vi "Obtain Module Semaphore.vi"(8 "error in":errorcluster) -> (0 "error out":errorcluster, 1 "created new?":bool, 3 "semaphore":T1)   [LabVIEW 2020, in "Camera Acquisition.lvlib"]
doc: "Obtain this module's Semaphore that locks down operations on the Clone Registry and VI Reference action engines.\n_____\nBased on DQMH Project Template 6.0.0.91."
uses:
  Camera Acquisition.lvlib
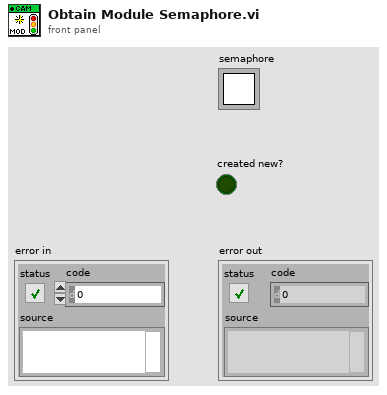
[diagram p1: front panel]
types:
  T1 = typedef "Semaphore RefNum" = refnum<k1>
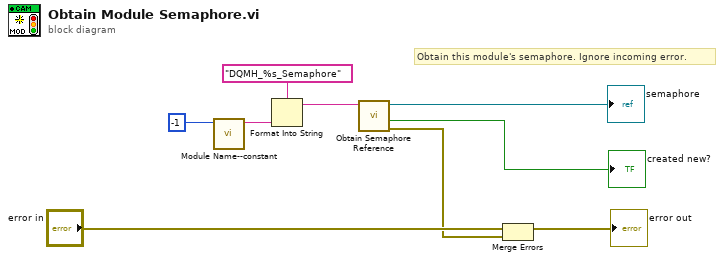
[diagram p0: block diagram]
diagram:
  # "Obtain this module's semaphore. Ignore incoming error."
  n1 = call "Module Name--constant.vi"("Module ID"=-1) -> ("Module Name"=w4:string)  [unwired: 10 in]
  n2 = Format Into String(format string="DQMH_%s_Semaphore", w4) -> (resulting string=w3:string)  [unwired: 2 in, 1 out]
  n3 = call <vilib>:"Obtain Semaphore Reference.vi"("name (unnamed)"=w3) -> ("error out"=w8:errorcluster, "created new"=→"created new?":bool, "semaphore"=→"semaphore":T1)  [unwired: 4 in]
  n4 = Merge Errors("error in", w8) -> (→"error out":errorcluster)
